vi "Range Logarithm Check.vi"(11 "Logarithm Range In":cluster{"Max":sgl, "Min":sgl}) -> (3 "Logarithm Range Out":cluster{"Max":sgl, "Min":sgl})   [LabVIEW 2020, in "3D Plot.lvclass"]
uses:
  <vilib>/Math Plots/3D Math Plots/3D Plot/3D Plot/3D Plot.lvclass
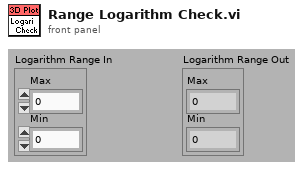
[diagram p1: front panel]
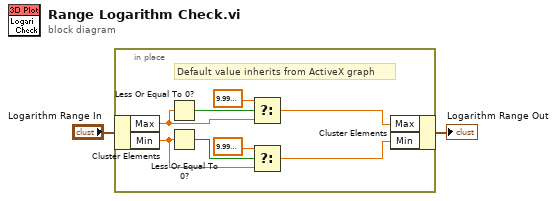
[diagram p0: block diagram]
diagram:
  n1 = in-place {
    # "Default value inherits from ActiveX graph"
    n2 = in-place-cluster #1("Logarithm Range In") -> ("Max"=w5:sgl, "Min"=w6:sgl)
    n3 = Less Or Equal To 0?(x=w5) -> (x <= 0?=w10:bool)
    n4 = Less Or Equal To 0?(x=w6) -> (x <= 0?=w9:bool)
    n5 = Select(t=sgl 0.0001 ("Min"), s=w10, f=w5) -> (s? t:f=w4:sgl)
    n6 = Select(t=sgl 1e-05 ("Min"), s=w9, f=w6) -> (s? t:f=w3:sgl)
    n7 = in-place-cluster #1("Max"=w4, "Min"=w3) -> (→"Logarithm Range Out":cluster{"Max":sgl, "Min":sgl})
  }
